vi "Launch Actor Core.vi"(8 "error in (no error)":errorcluster, 9 "Open Actor Core front panel?":bool, 10 "Caller's Enqueuer":refnum<class "Message Enqueuer.lvclass">, 11 "Actor in":refnum<class "Actor.lvclass">) -> (0 "error out":errorcluster, 3 "Message Enqueuer out":refnum<class "Message Enqueuer.lvclass">)   [LabVIEW 2014, in "Actor Framework.lvlib" / "Actor.lvclass"]
uses:
  <vilib>/ActorFramework/Actor/Actor.lvclass
  <vilib>/ActorFramework/Message Enqueuer/Message Enqueuer.lvclass
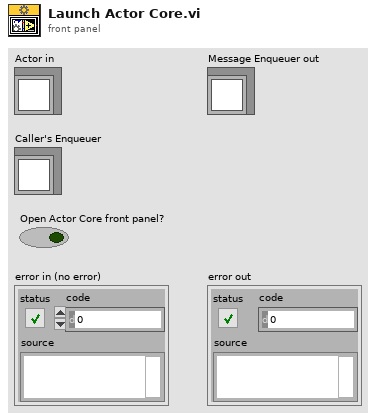
[diagram p1: front panel]
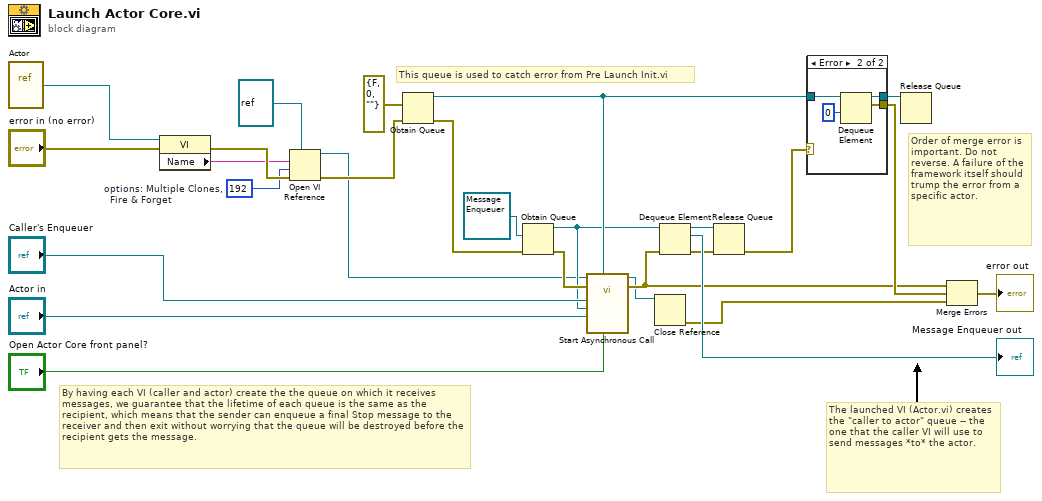
[diagram p0: block diagram]
diagram:
  w9 = 192  # options: Multiple Clones,   Fire & Forget
  # "By having each VI (caller and actor) create the the queue on which it receives messages, we guarantee that the lifetime of each queue is the same as the recipient, which means that the sender can enqueue a final Stop message to the receiver and then exit without worrying that the queue will be destroyed before the recipient gets the message."
  # "This queue is used to catch error from Pre Launch Init.vi"
  # "Order of merge error is important. Do not reverse. A failure of the framework itself should trump the error from a specific actor."
  # "The launched VI (Actor.vi) creates the \"caller to actor\" queue -- the one that the caller VI will use to send messages *to* the actor."
  n1 = vi-ref <vilib>:"Actor.vi"() -> (w8:refnum<vi>)
  n2 = property class="VI"(reference=w8, error in="error in (no error)") -> (error out=w11:errorcluster, "Name"=w10:string)  [unwired: 1 out]
  n3 = Open VI Reference(type specifier VI Refnum (for type only)=refnum<vi> refnum, vi path=w10, options=w9, error in (no error)=w11) -> (vi reference=w4:refnum<vi>, error out=w5:errorcluster)  [unwired: 2 in]
  n4 = Obtain Queue(element data type=errorcluster {"status"=FALSE, "code"=0, "source"=""} ("Error"), error in (no error)=w5) -> (queue out=w22:refnum<queue>, error out=w20:errorcluster)  [unwired: 3 in, 1 out]
  n5 = Obtain Queue(element data type=refnum<class "Message Enqueuer.lvclass"> refnum ("Message Enqueuer"), error in (no error)=w20) -> (queue out=w17:refnum<queue>, error out=w26:errorcluster)  [unwired: 3 in, 1 out]
  n6 = call-by-ref "Start Asynchronous Call"(reference=w4, error in=w26, "Open Actor Core front panel? (F)"="Open Actor Core front panel?", "error feedback"=w22, "Actor"="Actor in", "queue of queues"=w17, "Send Queue"="Caller's Enqueuer") -> (reference out=w3:refnum<vi>, error out=w7:errorcluster)  [unwired: 7 in]
  n7 = Close Reference(reference=w3) -> (error out=w2:errorcluster)  [unwired: 1 in]
  n8 = Dequeue Element(queue=w17, error in (no error)=w7) -> (queue out=w13:refnum<queue>, element=→"Message Enqueuer out":refnum<class "Message Enqueuer.lvclass">, error out=w14:errorcluster)  [unwired: 1 in, 1 out]
  n9 = Release Queue(queue=w13, error in (no error)=w14) -> (error out=w24:errorcluster)  [unwired: 1 in, 2 out]
  n10 = case shown="Error" w24 {
    selector: w24 -> [w29 _]
    tunnel: w22 -> [w28 w33]
    tunnel: [w29 w31] -> w23
    tunnel: [w28 w30] -> w25
    frame No Error {
    }
    frame Error {
      n11 = Dequeue Element(queue=w33, timeout in ms (-1)=0) -> (queue out=w30:refnum<queue>, element=w31:errorcluster)  [unwired: 1 in, 2 out]
    }
  }
  n12 = Release Queue(queue=w25) -> ()  [unwired: 2 in, 3 out]
  n13 = Merge Errors(w7, w23, w2) -> (→"error out":errorcluster)
